vi "setCommunicator.vi"(10 "Communicator":refnum<class "Communicator.lvclass">, 11 "Publisher in":refnum<class "Publisher.lvclass">) -> (3 "Publisher out":refnum<class "Publisher.lvclass">)   [LabVIEW 2016, in "Publisher.lvclass"]
uses:
  Publisher.lvclass
  Communicator/Communicator/Communicator.lvclass
  Publisher.lvclass/Publisher.ctl
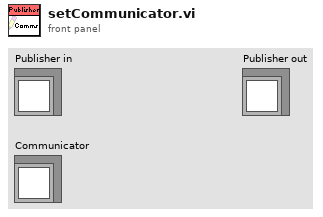
[diagram p1: front panel]
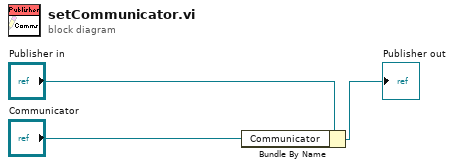
[diagram p0: block diagram]
diagram:
  n1 = Bundle By Name(cluster="Publisher in", "Communicator"="Communicator") -> (→"Publisher out":refnum<class "Publisher.lvclass">)
